vi "Create Messages.vi"(8 "error in (no error)":errorcluster, 10 "Initialize?":bool, 11 "Engine Data in":T2) -> (0 "error out":errorcluster, 1 "Connect Messages":T1[](array[typedef]), 2 "Disconnect Messages":T1[](array[typedef]), 3 "Engine Data out":T2)   [LabVIEW 2020, in "Routing and Faulting Engine.lvlib"]
uses:
  Routing and Faulting Engine.lvlib
  Engine Data.ctl
  Includes/CDMessaging.lvlibp/Producer/Abstract Producer/Abstract Producer.lvclass
  Shared/Compiled.Settings.ctl
  Shared/Communication Configuration.ctl
  Shared/Routing and Faulting Configuration.ctl
  Shared/Routing Channel Configuration.ctl
  Shared/Value-Connections Map.ctl
  Shared/Alias Mapping.ctl
  Shared/Alias Endpoint.ctl
  Shared/Compiled Connection.ctl
  Shared/FIFO Indices.ctl
  Device Inputs.ctl
  Device Outputs.ctl
  Producer Message.ctl
  Includes/CDMessaging.lvlibp/Message/Abstract Message/Abstract Message.lvclass
  f117cfd3-3adc-40fc-b63f-36de5ebdde45.vi
  3305a376-d4c0-444a-b726-8088d0367693.vi
  Shared/Get State Value Index.vi
  Shared/Convert State Value to Integer.vi
  Includes/CDMessaging.lvlibp/Switch/Switch Disconnect Message/Switch Disconnect Message.lvclass
  C:/Users/mjacobso/Desktop/SCM/Routing-Faulting/Includes/CDMessaging.lvlibp/Message/Abstract Request Message/Abstract Request Message.lvclass
  Includes/CDMessaging.lvlibp/Message/Abstract Request Message/Abstract Request Message.lvclass
  C:/Users/mjacobso/Desktop/SCM/Routing-Faulting/Includes/CDMessaging.lvlibp/Message/Abstract Message/Abstract Message.lvclass
  Includes/CDMessaging.lvlibp/Switch/Switch Connect Message/Switch Connect Message.lvclass
  <vilib>/Utility/error.llb/Error Cluster From Error Code.vi
  Shared/Routing and Faulting Shared.lvlib
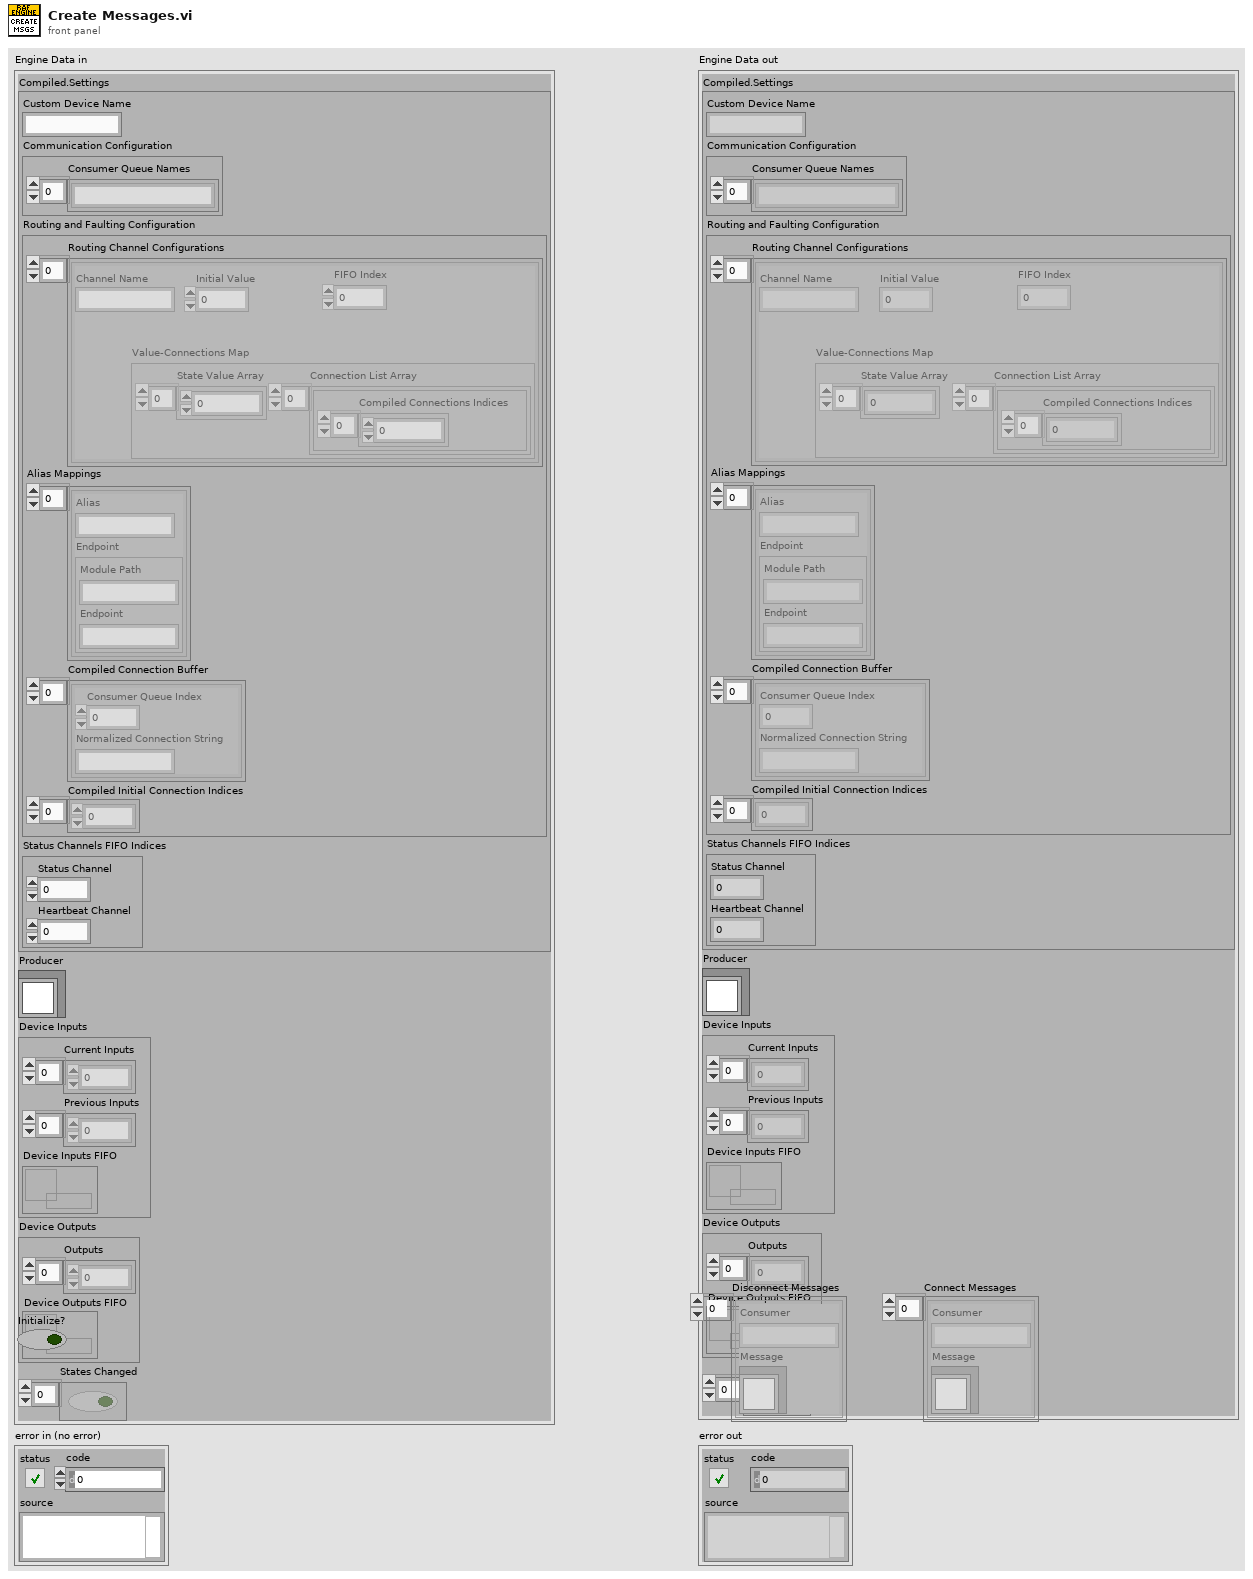
[diagram p1: front panel]
types:
  T1 = typedef "Routing and Faulting Engine.lvlib/Producer Message.ctl" = cluster{"Consumer":string, "Message":refnum<class "Abstract Message.lvclass">}
  T2 = typedef "Routing and Faulting Engine.lvlib/Engine Data.ctl" = cluster{"Compiled.Settings":T3, "Producer":refnum<class "Abstract Producer.lvclass">, "Device Inputs":T12, "Device Outputs":T13, "States Changed":bool[]}
  T3 = typedef "Routing and Faulting Shared.lvlib/Compiled.Settings.ctl" = cluster{"Custom Device Name":string, "Communication Configuration":T4, "Routing and Faulting Configuration":T5, "Status Channels FIFO Indices":T11}
  T4 = typedef "Routing and Faulting Shared.lvlib/Communication Configuration.ctl" = cluster{"Consumer Queue Names":string[]}
  T5 = typedef "Routing and Faulting Shared.lvlib/Routing and Faulting Configuration.ctl" = cluster{"Routing Channel Configurations":T6[], "Alias Mappings":T8[], "Compiled Connection Buffer":T10[], "Compiled Initial Connection Indices":i32[]}
  T6 = typedef "Routing and Faulting Shared.lvlib/Routing Channel Configuration.ctl" = cluster{"Channel Name":string, "Initial Value":dbl, "FIFO Index":i32, "Value-Connections Map":T7}
  T7 = typedef "Routing and Faulting Shared.lvlib/Value-Connections Map.ctl" = cluster{"State Value Array":i32[], "Connection List Array":cluster{"Compiled Connections Indices":i32[]}[]}
  T8 = typedef "Routing and Faulting Shared.lvlib/Alias Mapping.ctl" = cluster{"Alias":string, "Endpoint":T9}
  T9 = typedef "Routing and Faulting Shared.lvlib/Alias Endpoint.ctl" = cluster{"Module Path":string, "Endpoint":string}
  T10 = typedef "Routing and Faulting Shared.lvlib/Compiled Connection.ctl" = cluster{"Consumer Queue Index":i32, "Normalized Connection String":string}
  T11 = typedef "Routing and Faulting Shared.lvlib/FIFO Indices.ctl" = cluster{"Status Channel":i32, "Heartbeat Channel":i32}
  T12 = typedef "Routing and Faulting Engine.lvlib/Device Inputs.ctl" = cluster{"Current Inputs":dbl[], "Previous Inputs":dbl[], "Device Inputs FIFO":refnum<k33>}
  T13 = typedef "Routing and Faulting Engine.lvlib/Device Outputs.ctl" = cluster{"Outputs":dbl[], "Device Outputs FIFO":refnum<k33>}
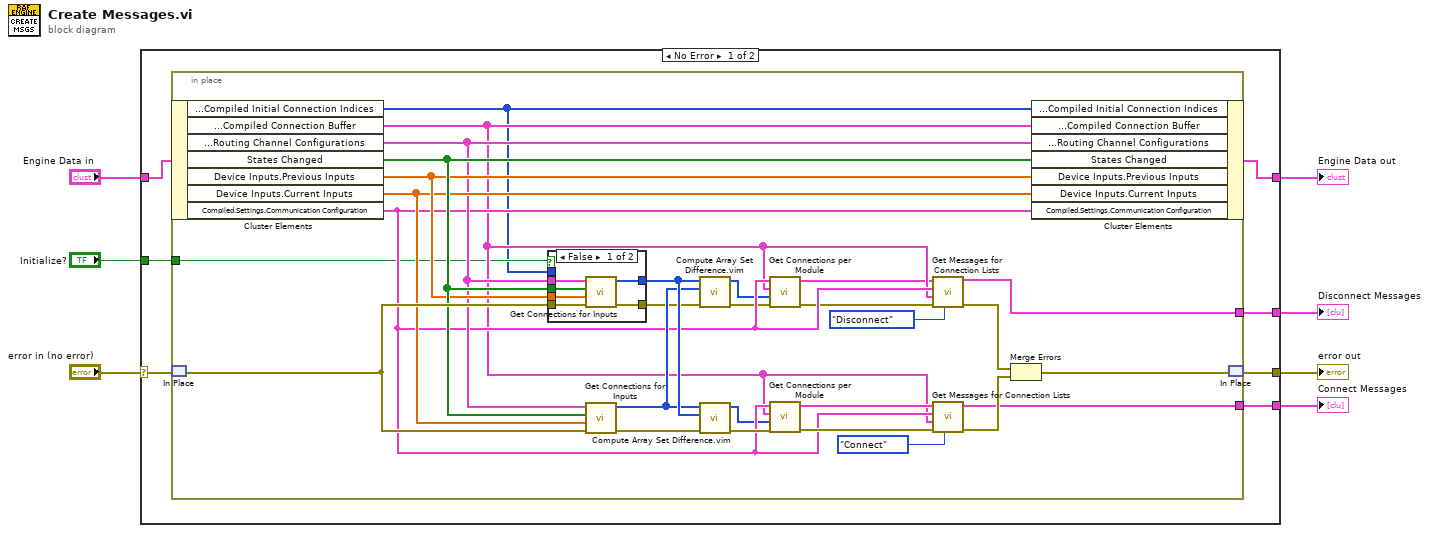
[diagram p0: block diagram]
diagram:
  n1 = case shown="No Error" "error in (no error)" {
    selector: "error in (no error)" -> [w14 w52]
    tunnel: "Engine Data in" -> [w10 w51]
    tunnel: [w13 w52] -> w5
    tunnel: [w12 w51] -> w4
    tunnel: [w11 _] -> w3
    tunnel: [w9 _] -> w2
    tunnel: "Initialize?" -> [w8 _]
    frame No Error {
      n2 = in-place {
        in-place-border: [w42] -> w11
        in-place-border: [w28] -> w9
        in-place-border: w8 -> [w16]
        n3 = in-place-cluster #1(w10) -> ("Compiled.Settings.Routing and Faulting Configuration.Compiled Initial Connection Indices"=w15:i32[], "Compiled.Settings.Routing and Faulting Configuration.Compiled Connection Buffer"=w24:T10[], "Compiled.Settings.Routing and Faulting Configuration.Routing Channel Configurations"=w27:T6[], "States Changed"=w40:bool[], "Device Inputs.Previous Inputs"=w33:dbl[], "Device Inputs.Current Inputs"=w32:dbl[], "Compiled.Settings.Communication Configuration"=w26:T4)
        n4 = in-place-match #2(w14) -> (w41:errorcluster)
        n5 = case shown="False" w16 {
          tunnel: w41 -> [w48 w49]
          tunnel: w40 -> [w47 _]
          tunnel: [w46 w50] -> w39
          tunnel: w33 -> [w45 _]
          tunnel: w27 -> [w44 _]
          tunnel: [w43 w49] -> w22
          tunnel: w15 -> [_ w50]
          frame False {
            n6 = call "Get Connections for Inputs.vi"("error in (no error)"=w48, "Inputs"=w45, "States Changed"=w47, "Routing Channel Configurations"=w44) -> ("error out"=w43:errorcluster, "Compiled Connections Indices"=w46:i32[])  [unwired: 6 in]
          }
          frame True {
          }
        }
        n7 = call "Get Connections for Inputs.vi"("error in (no error)"=w41, "Inputs"=w32, "States Changed"=w40, "Routing Channel Configurations"=w27) -> ("error out"=w37:errorcluster, "Compiled Connections Indices"=w38:i32[])  [unwired: 6 in]
        n8 = call "Compute Array Set Difference.vim"("error in (no error)"=w22, "B"=w38, "A"=w39) -> ("error out"=w19:errorcluster, "A - B"=w17:i32[])  [unwired: 7 in]
        n9 = call "Compute Array Set Difference.vim"("error in (no error)"=w37, "B"=w39, "A"=w38) -> ("error out"=w34:errorcluster, "A - B"=w25:i32[])  [unwired: 7 in]
        n10 = call "Get Connections per Module.vi"("error in (no error)"=w19, "Compiled Connections Indices"=w17, "Compiled Connection Buffer"=w24, "Communication Configuration"=w26) -> ("error out"=w20:errorcluster, "Connection Lists for each Module"=w21:cluster{"Indices":i32[]}[])  [unwired: 6 in]
        n11 = call "Get Connections per Module.vi"("error in (no error)"=w34, "Compiled Connections Indices"=w25, "Compiled Connection Buffer"=w24, "Communication Configuration"=w26) -> ("error out"=w36:errorcluster, "Connection Lists for each Module"=w35:cluster{"Indices":i32[]}[])  [unwired: 6 in]
        n12 = call "Get Messages for Connection Lists.vi"("Message Type"=enum16{"Connect", "Disconnect"}."Disconnect", "error in (no error)"=w20, "Compiled Connection Buffer"=w24, "Communication Configuration"=w26, "Connection Lists for each Module"=w21) -> ("error out"=w31:errorcluster, "Messages"=w42:T1[])  [unwired: 5 in]
        n13 = call "Get Messages for Connection Lists.vi"("Message Type"=enum16{"Connect", "Disconnect"}."Connect", "error in (no error)"=w36, "Compiled Connection Buffer"=w24, "Communication Configuration"=w26, "Connection Lists for each Module"=w35) -> ("error out"=w30:errorcluster, "Messages"=w28:T1[])  [unwired: 5 in]
        n14 = Merge Errors(w31, w30) -> (w29:errorcluster)
        n15 = in-place-cluster #1("Compiled.Settings.Routing and Faulting Configuration.Compiled Initial Connection Indices"=w15, "Compiled.Settings.Routing and Faulting Configuration.Compiled Connection Buffer"=w24, "Compiled.Settings.Routing and Faulting Configuration.Routing Channel Configurations"=w27, "States Changed"=w40, "Device Inputs.Previous Inputs"=w33, "Device Inputs.Current Inputs"=w32, "Compiled.Settings.Communication Configuration"=w26) -> (w12:T2)
        n16 = in-place-match #2(w29) -> (w13:errorcluster)
      }
    }
    frame Error {
    }
  }
  "Engine Data out" <- w4
  "error out" <- w5
  "Disconnect Messages" <- w3
  "Connect Messages" <- w2
